vi "WriteCAlexFile.vi"(6 "Overwrite?(F)":bool, 8 "error in (no error)":errorcluster, 10 "Output Path":path, 11 "CAlexData":refnum<class "CAlex2_Data.lvclass">) -> (0 "error out":errorcluster, 1 "Actual File Name":string, 2 "Output Path dup":path, 3 "CAlexData 2":refnum<class "CAlex2_Data.lvclass">)   [LabVIEW 2016, in "CAlex2_Data.lvclass"]
uses:
  CAlex2_Data.lvclass
  C:/Users/randh/Desktop/CABLE-LABVIEW/CALEX/CAlex2-controller/Sim&Process/DataProcess/ExpData/ExpData.lvclass
  CAlex2_Data.lvclass/CAlex2_Data.ctl
  ExpData/ExpData.lvclass
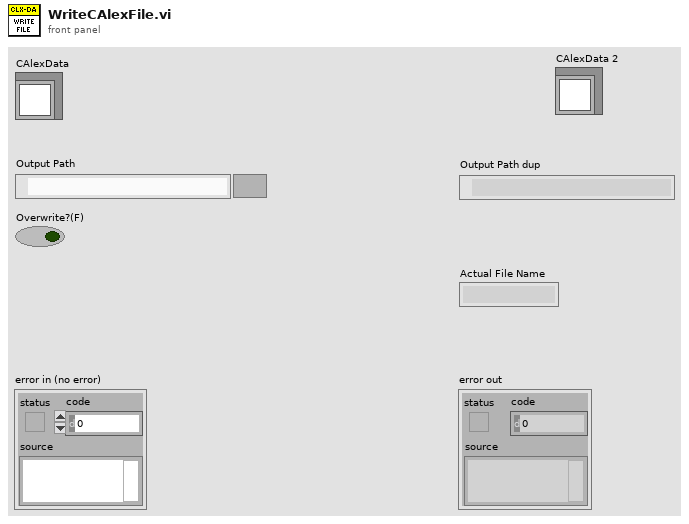
[diagram p1: front panel]
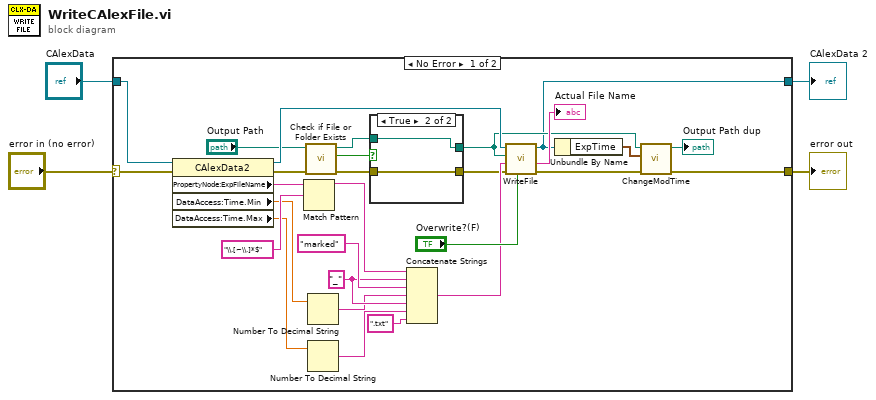
[diagram p0: block diagram]
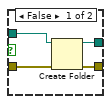
[diagram p2: hidden frame]
diagram:
  n1 = case shown="No Error" "error in (no error)" {
    selector: "error in (no error)" -> [w28 w40]
    tunnel: [w13 w40] -> w3
    tunnel: [w16 w39] -> w1
    tunnel: "CAlexData" -> [w30 w39]
    frame No Error {
      w8 = "_" ("string")
      n2 = property class="CAlexData2"(reference=w30, error in=w28) -> (reference out=w29:refnum<class "CAlex2_Data.lvclass">, error out=w22:errorcluster, "PropertyNode:ExpFileName"=w12:string, "DataAccess:Time.Min"=w10:dbl, "DataAccess:Time.Max"=w6:dbl)
      n3 = Match Pattern(string=w12, regular expression="\\.[~\\.]*$") -> (before substring=w19:string)  [unwired: 4 out]
      n4 = call <vilib>:"Check if File or Folder Exists.vi"("error in (no error)"=w22, "path"="Output Path") -> ("error out"=w25:errorcluster, "file or folder exists?"=w26:bool, "dup path"=w24:path)  [unwired: 7 in]
      n5 = Number To Decimal String(number=w10) -> (decimal integer string=w7:string)  [unwired: 1 in]
      n6 = Number To Decimal String(number=w6) -> (decimal integer string=w5:string)  [unwired: 1 in]
      n7 = case shown="True" w26 {
        tunnel: [w36 w38] -> w18
        tunnel: [w35 w37] -> w23
        tunnel: w24 -> [w34 w38]
        tunnel: w25 -> [w33 w37]
        frame False {
          n8 = Create Folder(path (use dialog)=w34, error in=w33) -> (created path=w36:path, error out=w35:errorcluster)  [unwired: 1 in, 1 out]
        }
        frame True {
        }
      }
      n9 = Concatenate Strings(w19, w8, "marked" ("string"), w7, w8, w5, ".txt" ("string")) -> (w27:string)
      n10 = call "WriteFile.vi"("Overwrite?(F)"="Overwrite?(F)", "error in (no error)"=w23, "Proposed File Name"=w27, "Output Path"=w18, "CarexData In"=w29) -> ("error out"=w14:errorcluster, "Actual File Name"=→"Actual File Name":string, "CarexData Out"=w16:refnum<class "CAlex2_Data.lvclass">)  [unwired: 4 in]
      n11 = Unbundle By Name(w16) -> ("ExpTime"=w15:timestamp)
      n12 = call <vilib>:"ChangeModTime.vi"("error in (no error)"=w14, "Time Stamp"=w15, "path"=w18) -> ("error out"=w13:errorcluster, "path dup"=→"Output Path dup":path)  [unwired: 7 in]
    }
    frame Error {
    }
  }
  "error out" <- w3
  "CAlexData 2" <- w1
